vi "filter.vi"(8 "Ts":dbl, 9 "y2":dbl, 10 "y1":dbl, 11 "Tf":dbl) -> (2 "yf2":dbl, 3 "yf1":dbl)   [LabVIEW 2019]
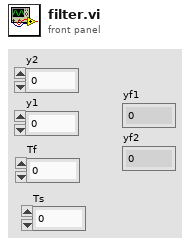
[diagram p1: front panel]
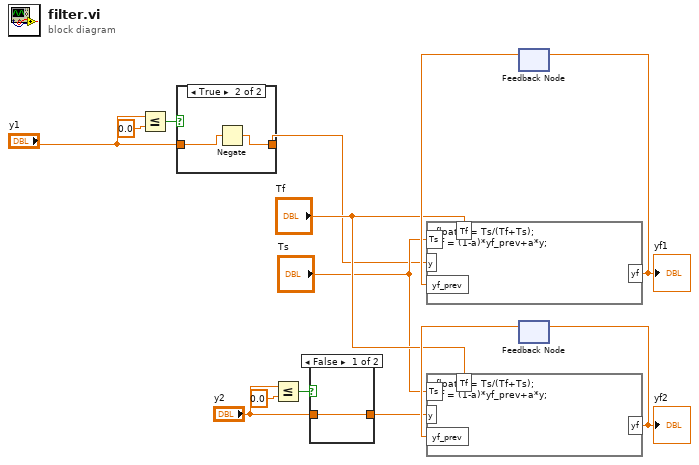
[diagram p0: block diagram]
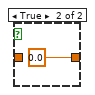
[diagram p3: hidden frame]
diagram:
  n1 = Less Or Equal?(x="y1", y=0.0) -> (x <= y?=w3:bool)
  n2 = case shown="True" w3 {
    tunnel: [w15 w17] -> w1
    tunnel: "y1" -> [w15 w16]
    frame False {
    }
    frame True {
      n3 = Negate(x=w16) -> (-x=w17:dbl)
    }
  }
  n4 = Less Or Equal?(x="y2", y=0.0) -> (x <= y?=w8:bool)
  n5 = case shown="False" w8 {
    tunnel: [w18 0.0] -> w6
    tunnel: "y2" -> [w18 _]
    frame False {
    }
    frame True {
    }
  }
  n6 = feedback #1() -> (w14:dbl)  [unwired: 1 in]
  n7 = formula code="float a = Ts/(Tf+Ts);\nyf = (1-a)*yf_prev+a*y;"("Tf"="Tf", "Ts"="Ts", "y"=w1, "yf_prev"=w14) -> ("yf"=w12:dbl)
  "yf1" <- w12
  n8 = feedback-in #1(w12) -> ()
  n9 = feedback #2() -> (w13:dbl)  [unwired: 1 in]
  n10 = formula code="float a = Ts/(Tf+Ts);\nyf = (1-a)*yf_prev+a*y;"("Tf"="Tf", "Ts"="Ts", "y"=w6, "yf_prev"=w13) -> ("yf"=w11:dbl)
  "yf2" <- w11
  n11 = feedback-in #2(w11) -> ()
